vi "InstrumentsList.vi"(8 "error in (no error)":errorcluster, 11 "ByteGSAPIBase in":refnum<class "ByteQXAPIBase.lvclass">) -> (0 "error out":errorcluster, 2 "Array":T1[](array[typedef]), 3 "ByteGSAPIBase out":refnum<class "ByteQXAPIBase.lvclass">)   [LabVIEW 2019, in "ByteQXWebAPI.lvlib" / "ByteQXAPIBase.lvclass"]
uses:
  ByteQXAPIBase.lvclass
  Instruments.ctl
  Private/module.ctl
  ByteQXAPIBase.lvclass/ByteQXAPIBase.ctl
  <vilib>/Bytelabs/ByteREST/ByteRESTClass/ByteRESTBase/RESTBase.lvclass
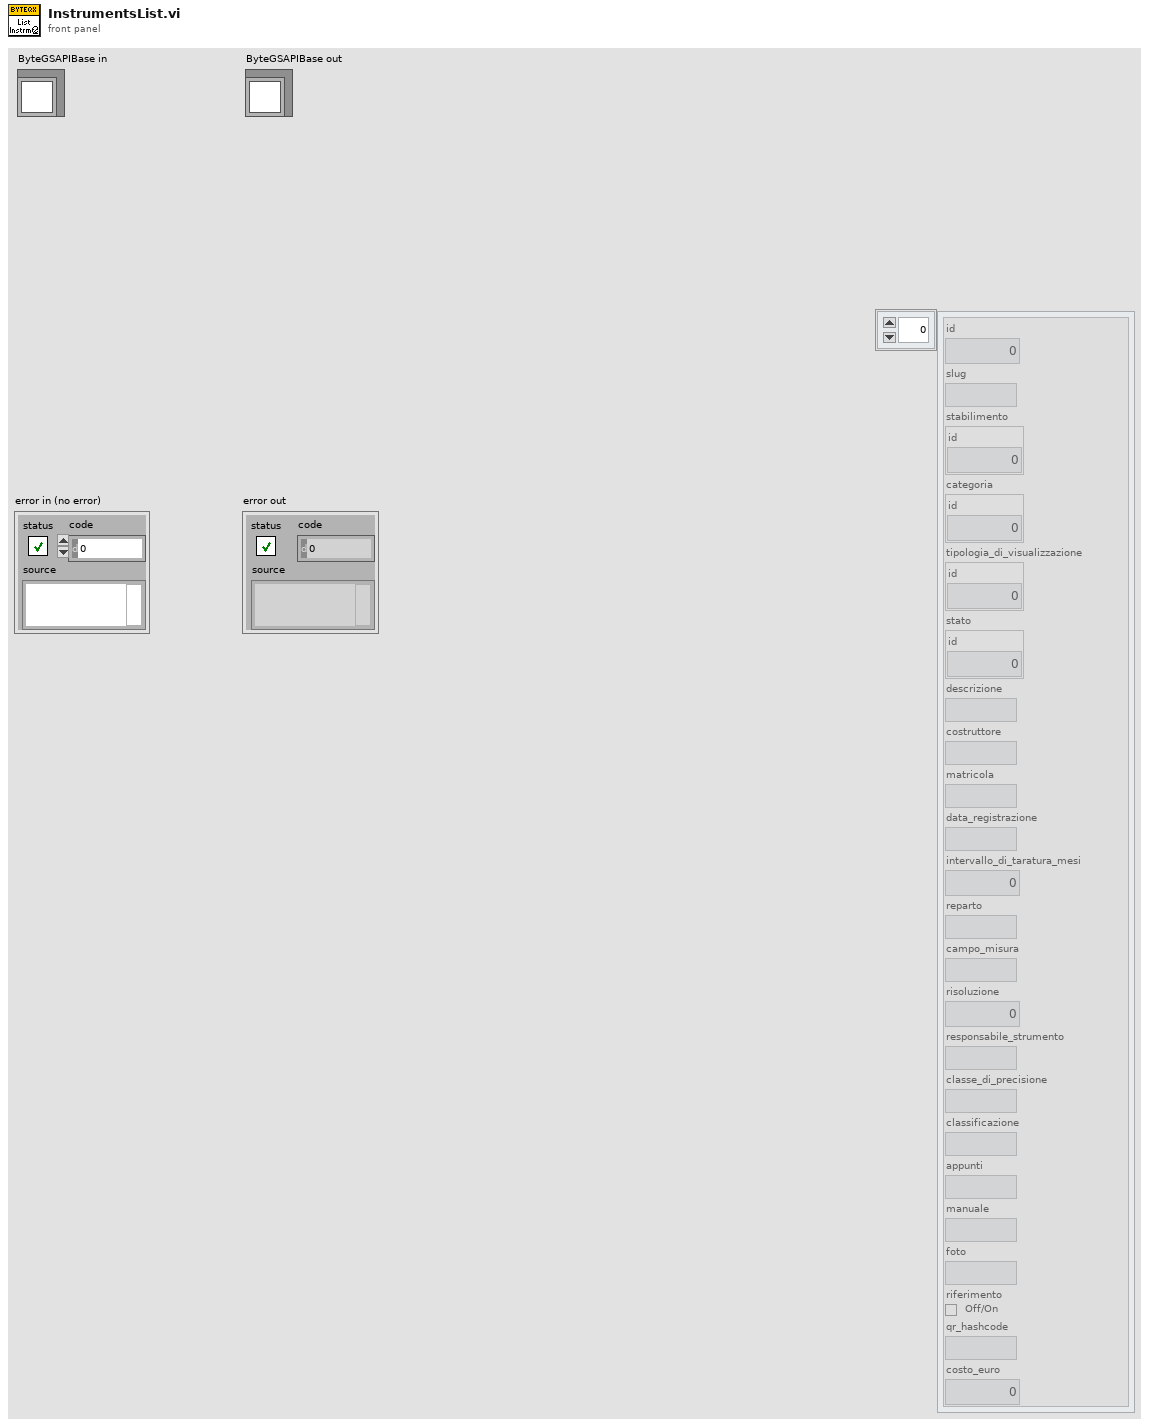
[diagram p1: front panel]
types:
  T1 = typedef "Instruments.ctl" = cluster{"id":i32, "slug":string, "stabilimento":cluster{"id":dbl}, "categoria":cluster{"id":dbl}, "tipologia_di_visualizzazione":cluster{"id":dbl}, "stato":cluster{"id":dbl}, "descrizione":string, "costruttore":string, "matricola":string, "data_registrazione":string, "intervallo_di_taratura_mesi":dbl, "reparto":string, "campo_misura":string, "risoluzione":dbl, "responsabile_strumento":string, "classe_di_precisione":string, "classificazione":string, "appunti":string, "manuale":string, "foto":string, "riferimento":bool, "qr_hashcode":string, "costo_euro":dbl}
  T2 = typedef "ByteQXWebAPI.lvlib/ByteQXAPIBase.lvclass/module.ctl" = enum16{"gs", "tms"}
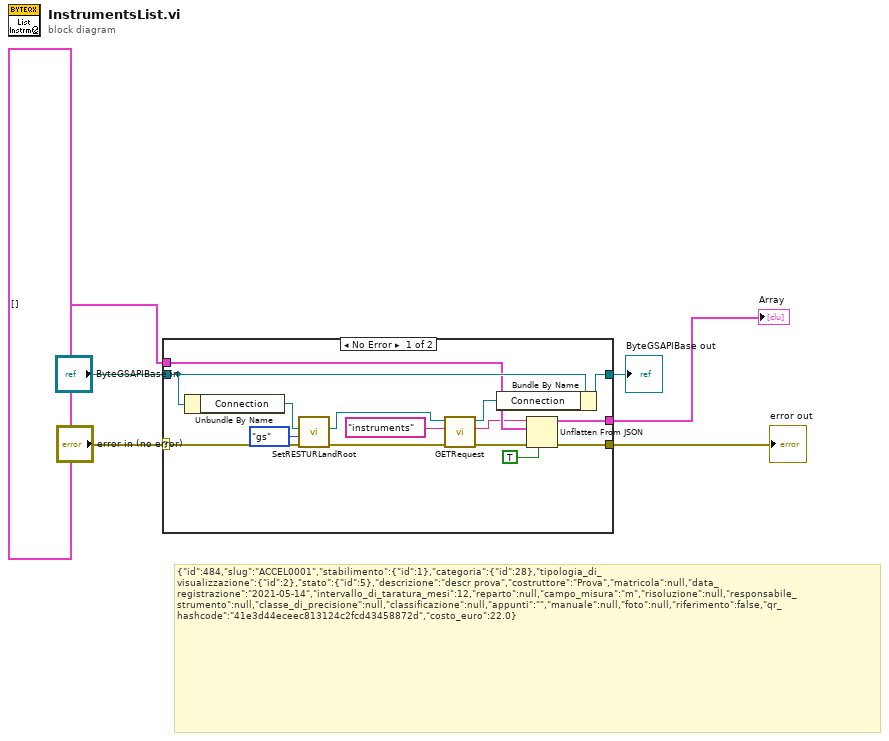
[diagram p0: block diagram]
diagram:
  # "{\"id\":484,\"slug\":\"ACCEL0001\",\"stabilimento\":{\"id\":1},\"categoria\":{\"id\":28},\"tipologia_di_visualizzazione\":{\"id\":2},\"stato\":{\"id\":5},\"descrizione\":\"descr prova\",\"costruttore\":\"Prova\",\"matricola\":null,\"data_registrazione\":\"2021-05-14\",\"intervallo_di_taratura_mesi\":12,\"reparto\":null,\"campo_misura\":\"m\",\"risoluzione\":null,\"responsabile_strumento\":null,\"classe_di_precisione\":null,\"classificazione\":null,\"appunti\":\"\",\"manuale\":null,\"foto\":null,\"riferimento\":false,\"qr_hashcode\":\"41e3d44eceec813124c2fcd43458872d\",\"costo_euro\":22.0}"
  n1 = case shown="No Error" "error in (no error)" {
    selector: "error in (no error)" -> [w11 w24]
    tunnel: [w16 w24] -> w4
    tunnel: T1[] [] ("SingleInstrument") -> [w15 w23]
    tunnel: [w14 w23] -> w1
    tunnel: [w19 w22] -> w5
    tunnel: "ByteGSAPIBase in" -> [w21 w22]
    frame No Error {
      n2 = Unbundle By Name(w21) -> ("Connection"=w9:refnum<class "RESTBase.lvclass">)
      n3 = call "SetRESTURLandRoot.vi"("error in (no error)"=w11, "module"=module."gs", "ByteREST in"=w9) -> ("error out"=w10:errorcluster, "ByteREST out"=w8:refnum<class "RESTBase.lvclass">)  [unwired: 7 in]
      n4 = call-dynamic "GETRequest.vi"("error in (no error)"=w10, "Request"="instruments", "ByteRESTBase in"=w8) -> ("error out"=w20:errorcluster, "Body"=w13:string, "ByteRESTBase out"=w18:refnum<class "RESTBase.lvclass">)  [unwired: 5 in, 1 out]
      n5 = Bundle By Name(cluster=w21, "Connection"=w18) -> (w19:refnum<class "ByteQXAPIBase.lvclass">)
      n6 = Unflatten From JSON(JSON string=w13, type and defaults=w15, default null elements? (F)=TRUE, error in (no error)=w20) -> (value=w14:T1[], error out=w16:errorcluster)  [unwired: 3 in]
    }
    frame Error {
    }
  }
  "error out" <- w4
  "ByteGSAPIBase out" <- w5
  "Array" <- w1
